vi "DB_Create.vi"(8 "error in":errorcluster) -> (0 "error out":errorcluster, 3 "SQLite Connection":refnum<class "Connection.lvclass">)   [LabVIEW 2020]
doc: "Creates the database holding the car wash data."
uses:
  <vilib>/drjdpowell/SQLite Library/SQL Connection/Connection.lvclass
  <vilib>/drjdpowell/SQLite Library/SQL Connection/Open (path).vi
  <vilib>/drjdpowell/SQLite Library/SQL Connection/Open (string).vi
  <vilib>/AdvancedString/Path To Command Line String.vi
  <vilib>/drjdpowell/SQLite Library/SQL Connection/Execute SQL (Single Integer).vi
  <vilib>/drjdpowell/SQLite Library/SQLite.lvlib
panel:
  in  "Subfolder 2":string="Example1.db"
  in  "Subfolder":string="Example1.db"
  out "Application Directory":path
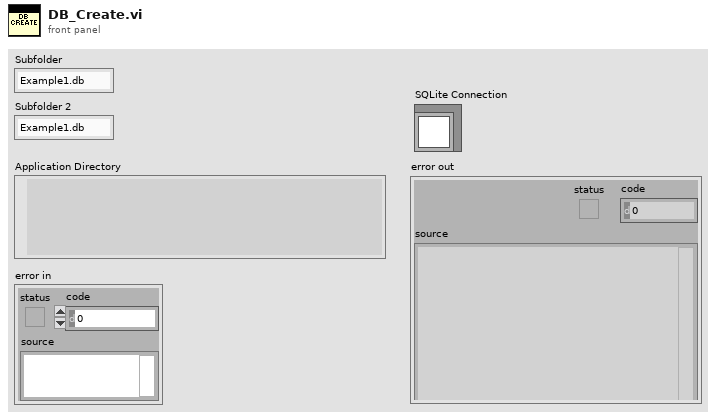
[diagram p1: front panel]
types:
  T1 = enum16{"New or existing", "Existing", "Read only"}
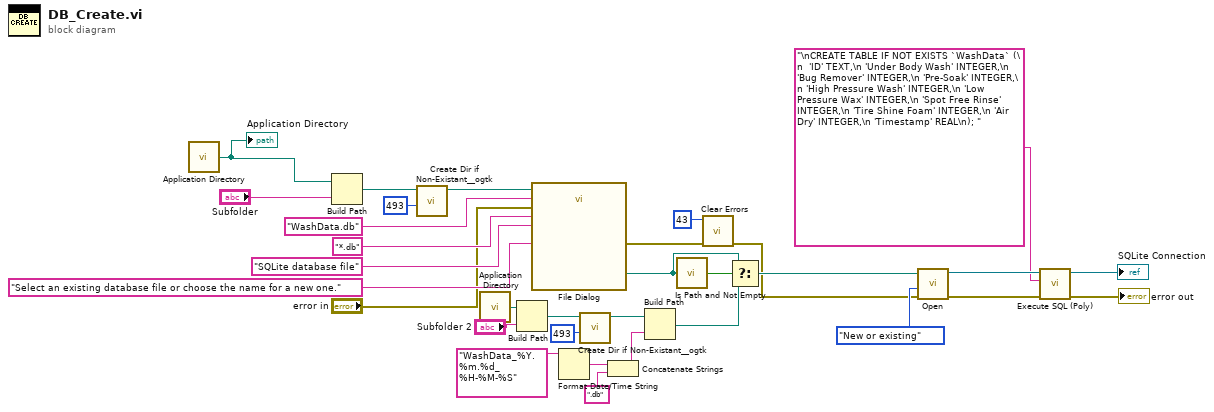
[diagram p0: block diagram]
diagram:
  n1 = call <vilib>:"Application Directory.vi"() -> ("Application Directory"=w27:path)
  "Application Directory" <- w27
  n2 = Build Path(base path=w27, name or relative path="Subfolder") -> (appended path=w6:path)
  n3 = call <userlib>:"Create Dir if Non-Existant__ogtk.vi"("permissions (0755)"=i16 493, "Directory Path"=w6) -> ("dup Directory Path"=w5:path)  [unwired: 7 in, 2 out]
  n4 = call <vilib>:"Application Directory.vi"() -> ("Application Directory"=w13:path)
  n5 = Build Path(base path=w13, name or relative path="Subfolder 2") -> (appended path=w2:path)
  n6 = call "File Dialog"("start path"=w5, "prompt"="Select an existing database file or choose the name for a new one.", "default name"="WashData.db", "error in"="error in", "pattern (all files)"="*.db", "pattern label"="SQLite database file") -> ("selected path"=w17:path, "error out"=w15:errorcluster)  [unwired: 6 in, 2 out]
  n7 = Format Date/Time String(time format string (%c)="WashData_%Y.%m.%d_%H-%M-%S") -> (date/time string=w10:string)  [unwired: 2 in]
  n8 = call <userlib>:"Create Dir if Non-Existant__ogtk.vi"("permissions (0755)"=i16 493, "Directory Path"=w2) -> ("dup Directory Path"=w3:path)  [unwired: 7 in, 2 out]
  n9 = Concatenate Strings(w10, ".db" ("string")) -> (w8:string)
  n10 = Build Path(base path=w3, name or relative path=w8) -> (appended path=w7:path)
  n11 = call <vilib>:"Is Path and Not Empty.vi"("path"=w17) -> ("Is Path and Not Empty?"=w20:bool)  [unwired: 4 in]
  n12 = call <vilib>:"Clear Errors.vi"("error in (no error)"=w15, "specific error code to clear (0: all)"=43) -> ("error out"=w14:errorcluster)  [unwired: 4 in, 1 out]
  n13 = Select(t=w17, s=w20, f=w7) -> (s? t:f=w18:path)
  n14 = call-poly <vilib>:"Open.vi"("error in (no error)"=w14, "File Option"=T1."New or existing", "db file"=w18) -> ("error out"=w29:errorcluster, "SQLite Connection"=w32:refnum<class "Connection.lvclass">)  [unwired: 7 in]
  n15 = call-poly <vilib>:"Execute SQL (Poly).vi"("error in (no error)"=w29, "SQL"="\nCREATE TABLE IF NOT EXISTS `WashData` (\n  'ID' TEXT,\n 'Under Body Wash' INTEGER,\n 'Bug Remover' INTEGER,\n 'Pre-Soak' INTEGER,\n 'High Pressure Wash' INTEGER,\n 'Low Pressure Wax' INTEGER,\n 'Spot Free Rinse' INTEGER,\n 'Tire Shine Foam' INTEGER,\n 'Air Dry' INTEGER,\n 'Timestamp' REAL\n); ", "SQLite Connection in"=w32) -> ("error out"=→"error out":errorcluster, "SQLite Connection"=→"SQLite Connection":refnum<class "Connection.lvclass">)  [unwired: 6 in, 1 out]
